vi "Get Address and Name Settings.vi"(8 "error in (no error)":errorcluster, 11 "Node Ref":T1 format="%.0x") -> (0 "error out":errorcluster, 2 "J1939 XNET Settings out":T2 {"Name" format="%.0x"}, 3 "Node Ref out":T1 format="%.0x")   [LabVIEW 2015, in "J1939 Addon System Explorer.lvlib"]
uses:
  J1939 Addon System Explorer.lvlib
  Shared/Types/Monitor Settings.ctl
  <vilib>/NI Veristand/Custom Device API/Custom Device Item Ref.ctl
  Shared/SubVIs/Constants.vi
  <vilib>/NI Veristand/Custom Device API/Get Item Property (Variant).vi
  <vilib>/NI VeriStand/Custom Device API/Custom Device API.lvlib
  Shared/J1939 Addon Shared.lvlib
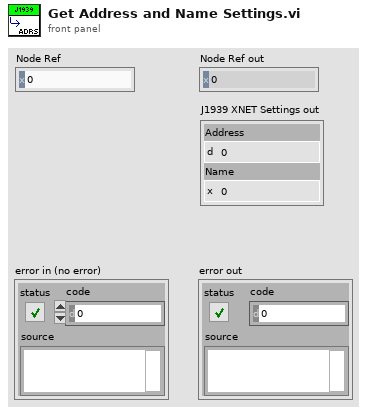
[diagram p1: front panel]
types:
  T1 = typedef "Custom Device API.lvlib/Custom Device Item Ref.ctl" = u64
  T2 = typedef "J1939 Addon Shared.lvlib/Monitor Settings.ctl" = cluster{"Address":u8, "Name":u64}
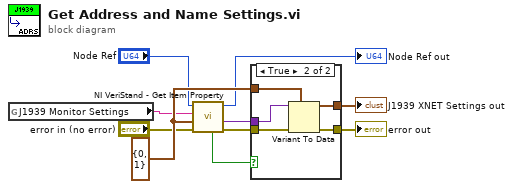
[diagram p0: block diagram]
diagram:
  w9 = T2 {"Address"=0, "Name"=1} ("J1939 XNET Settings in")
  n1 = global read "Constants.vi" "J1939 Monitor Settings"() -> (w1:string)
  n2 = call-poly <vilib>:"NI VeriStand - Get Item Property.vi"("error in (no error)"="error in (no error)", "Default Value"=w9, "Property Name"=w1, "Item Ref in"="Node Ref") -> ("error out"=w3:errorcluster, "Value"=w7:variant, "Item Ref out"=→"Node Ref out":T1, "Found?"=w8:bool)  [unwired: 4 in]
  n3 = case shown="True" w8 {
    tunnel: w3 -> [w12 w17]
    tunnel: [w12 w16] -> w6
    tunnel: w7 -> [_ w15]
    tunnel: w9 -> [w11 w14]
    tunnel: [w11 w13] -> w10
    frame False {
    }
    frame True {
      n4 = Variant To Data(error in=w17, type=w14, Variant=w15) -> (data=w13:T2, error out=w16:errorcluster)
    }
  }
  "J1939 XNET Settings out" <- w10
  "error out" <- w6
